vi "RT Loop Status.vi"(7 "Finished Late?":bool, 8 "error in (no error)":errorcluster, 9 "Loop Timeout in":u32, 10 "Finished Late Counter in":i32, 11 "Iteration Duration":i64) -> (0 "error out":errorcluster, 1 "Loop Timeout out":u32, 2 "Finished Late Counter out":i32, 3 "Loop Status":T1 {"Duration, us" format="%0.2f"})   [LabVIEW 2017]
doc: "Perform and prepare a staus data of RT Timed loop"
uses:
  RT Loop Status.ctl
  <vilib>/ptbypt/NI_PtbyPt.lvlib
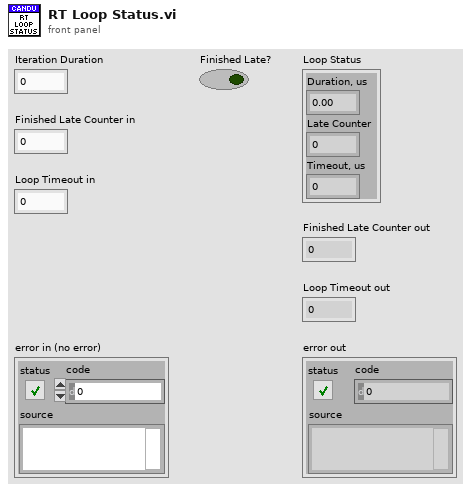
[diagram p1: front panel]
types:
  T1 = typedef "RT Loop Status.ctl" = cluster{"Duration, us":dbl, "Late Counter":i32, "Timeout, us":u32}
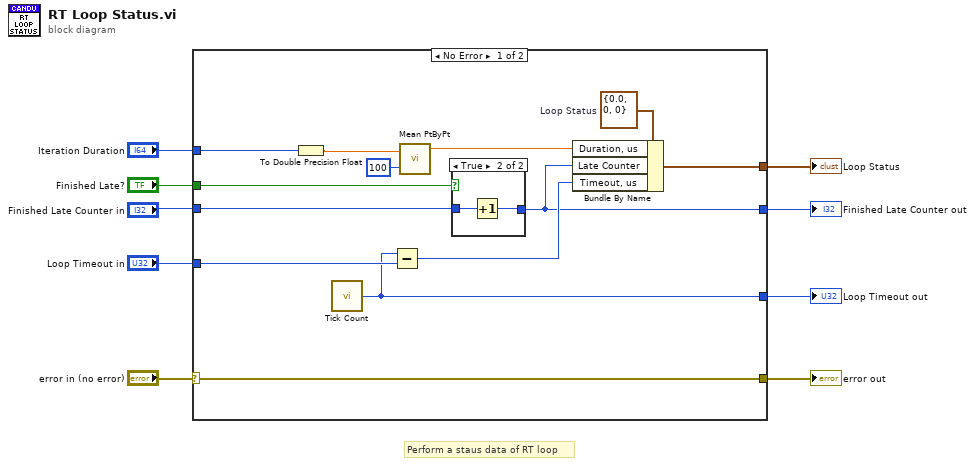
[diagram p0: block diagram]
diagram:
  # "Perform a staus data of RT loop"
  n1 = case shown="No Error" "error in (no error)" {
    selector: "error in (no error)" -> [w22 w26]
    tunnel: [w22 w26] -> w8
    tunnel: "Iteration Duration" -> [w16 _]
    tunnel: "Finished Late?" -> [w15 _]
    tunnel: "Finished Late Counter in" -> [w14 _]
    tunnel: "Loop Timeout in" -> [w13 _]
    tunnel: [w12 _] -> w3
    tunnel: [w11 _] -> w2
    tunnel: [w10 _] -> w1
    frame No Error {
      w19 = T1 {"Duration, us"=0.0, "Late Counter"=0, "Timeout, us"=0}  # Loop Status
      n2 = To Double Precision Float(number=w16) -> (double precision float=w18:dbl)
      n3 = call "Tick Count"() -> ("Tick Count(uSec)"=w12:u32)
      n4 = Subtract(x=w12, y=w13) -> (x-y=w17:u32)
      n5 = call <vilib>:"Mean PtByPt.vi"("x"=w18, "sample length"=100) -> ("mean"=w20:dbl)  [unwired: 2 in, 1 out]
      n6 = case shown="True" w15 {
        tunnel: w14 -> [w23 w25]
        tunnel: [w23 w24] -> w11
        frame False {
        }
        frame True {
          n7 = Increment(x=w25) -> (x+1=w24:i32)
        }
      }
      n8 = Bundle By Name(cluster=w19, "Duration, us"=w20, "Late Counter"=w11, "Timeout, us"=w17) -> (w10:T1)
    }
    frame Error {
    }
  }
  "error out" <- w8
  "Finished Late Counter out" <- w2
  "Loop Timeout out" <- w3
  "Loop Status" <- w1
